vi "Create Dictionary.vi"(7 "SMO.Dictionary":refnum<class "SMO.Dictionary.lvclass">, 8 "error in (no error)":errorcluster, 10 "Subsystem Name (optional)":string) -> (0 "error out":errorcluster, 2 "SMO name":string, 3 "SMO.Dictionary out":refnum<class "SMO.Dictionary.lvclass">)   [LabVIEW 2013, in "SMO.Dictionary.lvlib" / "SMO.Dictionary.lvclass"]
uses:
  SMO.Dictionary.lvclass
  <vilib>/JKI/JKI SMO/SMO/SMO.lvclass
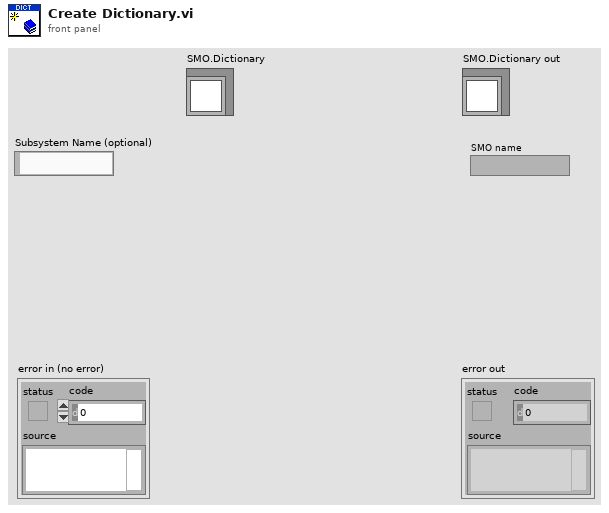
[diagram p1: front panel]
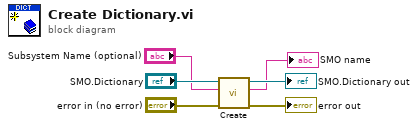
[diagram p0: block diagram]
diagram:
  n1 = call <vilib>:"Create.vi"("error in (no error)"="error in (no error)", "Subsystem Name (optional)"="Subsystem Name (optional)", "SMO"="SMO.Dictionary") -> ("error out"=→"error out":errorcluster, "SMO name"=→"SMO name":string, "SMO out"=→"SMO.Dictionary out":refnum<class "SMO.Dictionary.lvclass">)  [unwired: 6 in]
